vi "labview.vi"() -> ()   [LabVIEW 2021]
uses:
  40da32ed-f428-4d30-ba7b-34cf0621b097.vi
  <vilib>/Utility/file.llb/Read Delimited Spreadsheet (string).vi
  <vilib>/Comparison/Less/Less Functor/Less Functor.lvclass
panel:
  out "Buys Cumputer":string
  out "output cluster":T1
  in  "file path (dialog if empty)":path
  in  "K Value":dbl
  in  "Query Instance":T2
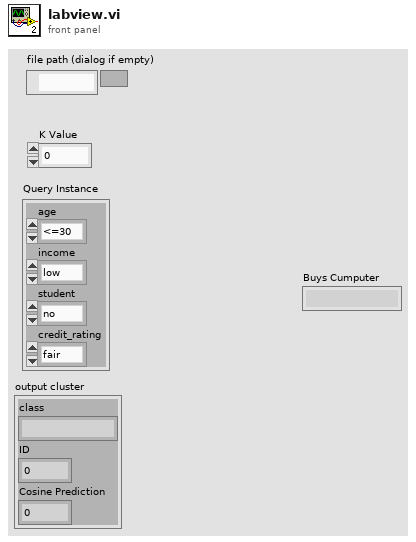
[diagram p1: front panel]
types:
  T1 = cluster{"class":string, "ID":dbl, "Cosine Prediction":dbl}
  T2 = cluster{"age":enum32{"<=30", "31...40", ">40"}, "income":enum32{"low", "medium", "high"}, "student":enum32{"no", "yes"}, "credit_rating":enum32{"fair", "excellent"}}
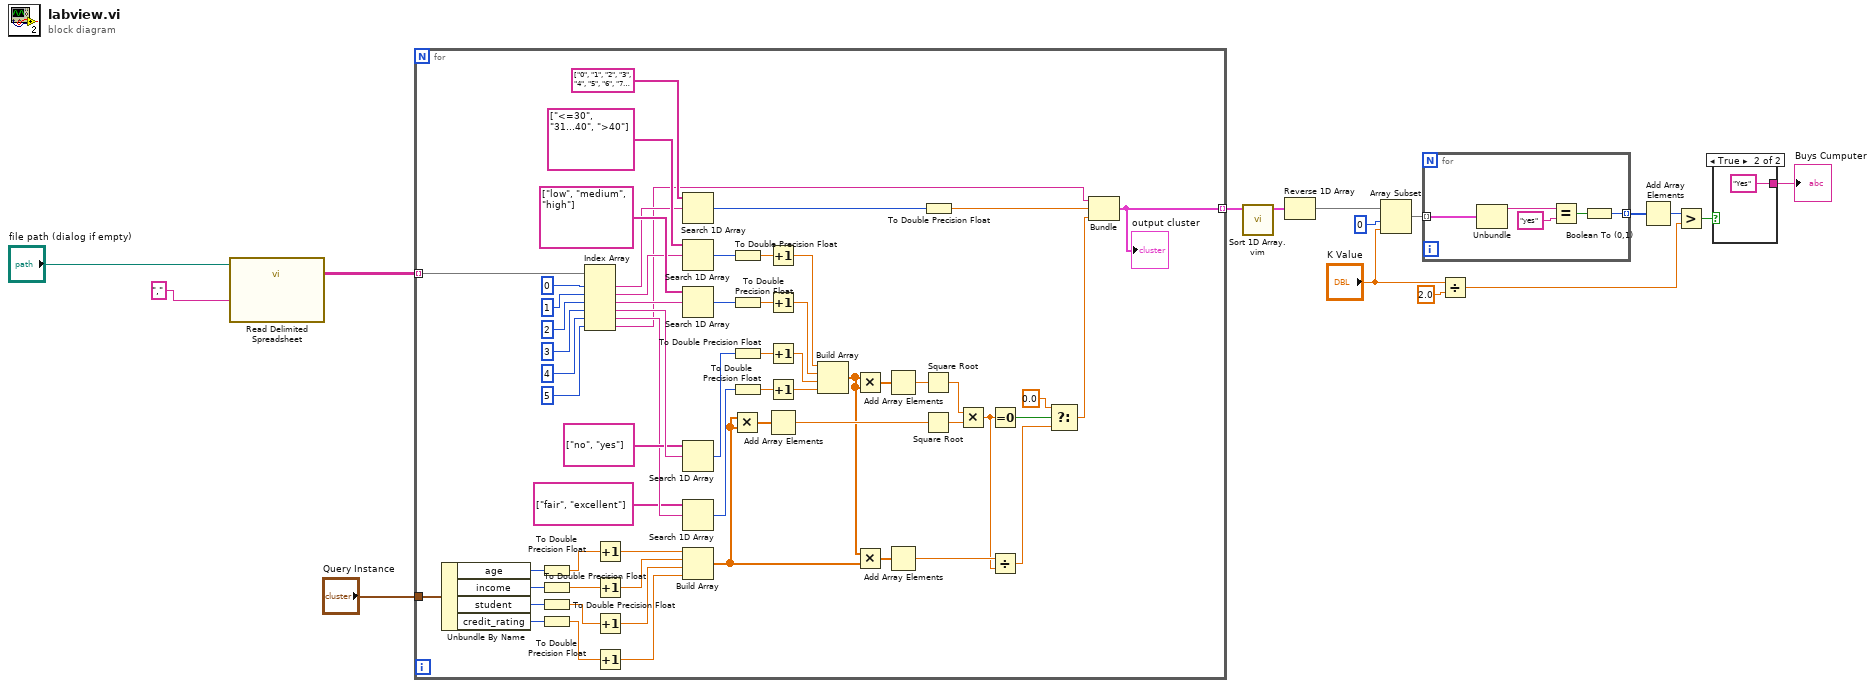
[diagram p0: block diagram]
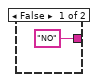
[diagram p2: hidden frame]
diagram:
  n1 = call-poly <vilib>:"Read Delimited Spreadsheet.vi"("file path (dialog if empty)"="file path (dialog if empty)", "delimiter (\\t)"="," ("delimiter (\\t)")) -> ("all rows"=w14:string[][])  [unwired: 8 in, 5 out]
  n2 = for {
    tunnel: w14 -> [w64] mode=indexing
    tunnel: "Query Instance" -> [w50]
    tunnel: [w24] -> w12 mode=indexing
    n3 = Unbundle By Name(w50) -> ("age"=w45:enum32{"<=30", "31...40", ">40"}, "income"=w44:enum32{"low", "medium", "high"}, "student"=w43:enum32{"no", "yes"}, "credit_rating"=w42:enum32{"fair", "excellent"})
    n4 = To Double Precision Float(number=w45) -> (double precision float=w49:dbl)
    n5 = To Double Precision Float(number=w44) -> (double precision float=w48:dbl)
    n6 = To Double Precision Float(number=w43) -> (double precision float=w47:dbl)
    n7 = To Double Precision Float(number=w42) -> (double precision float=w46:dbl)
    n8 = Index Array(array=w64, index #1=0 ("index"), index #2=1 ("index"), index #3=2 ("index"), index #4=3 ("index"), index #5=4 ("index"), index #6=5 ("index")) -> (element #1=w27:string, element #2=w70:string, element #3=w71:string, element #4=w68:string, element #5=w66:string, element #6=w18:string)
    n9 = Increment(x=w49) -> (x+1=w41:dbl)
    n10 = Increment(x=w48) -> (x+1=w40:dbl)
    n11 = Increment(x=w47) -> (x+1=w39:dbl)
    n12 = Increment(x=w46) -> (x+1=w38:dbl)
    n13 = Search 1D Array(1D array=string[] ["0", "1", "2", "3", "4", "5", "6", "7", "8", "9", "10", "11", "12", "13"], element=w27) -> (index of element=w26:i32)  [unwired: 1 in]
    n14 = Search 1D Array(1D array=string[] ["<=30", "31...40", ">40"], element=w70) -> (index of element=w62:i32)  [unwired: 1 in]
    n15 = Search 1D Array(1D array=string[] ["low", "medium", "high"], element=w71) -> (index of element=w59:i32)  [unwired: 1 in]
    n16 = Search 1D Array(1D array=string[] ["no", "yes"], element=w68) -> (index of element=w57:i32)  [unwired: 1 in]
    n17 = Search 1D Array(1D array=string[] ["fair", "excellent"], element=w66) -> (index of element=w55:i32)  [unwired: 1 in]
    n18 = Build Array(w41, w40, w39, w38) -> (w35:dbl[])
    n19 = Multiply(x=w35, y=w35) -> (x*y=w34:dbl[])
    n20 = To Double Precision Float(number=w62) -> (double precision float=w61:dbl)
    n21 = To Double Precision Float(number=w59) -> (double precision float=w60:dbl)
    n22 = To Double Precision Float(number=w57) -> (double precision float=w58:dbl)
    n23 = To Double Precision Float(number=w55) -> (double precision float=w56:dbl)
    n24 = Increment(x=w61) -> (x+1=w54:dbl)
    n25 = Increment(x=w60) -> (x+1=w53:dbl)
    n26 = Increment(x=w58) -> (x+1=w52:dbl)
    n27 = Increment(x=w56) -> (x+1=w51:dbl)
    n28 = Add Array Elements(numeric array=w34) -> (sum=w33:dbl)
    n29 = Build Array(w54, w53, w52, w51) -> (w29:dbl[])
    n30 = Multiply(x=w29, y=w29) -> (x*y=w32:dbl[])
    n31 = Multiply(x=w29, y=w35) -> (x*y=w37:dbl[])
    n32 = Add Array Elements(numeric array=w32) -> (sum=w31:dbl)
    n33 = Add Array Elements(numeric array=w37) -> (sum=w36:dbl)
    n34 = Square Root(x=w31) -> (sqrt(x)=w28:dbl)
    n35 = Square Root(x=w33) -> (sqrt(x)=w30:dbl)
    n36 = To Double Precision Float(number=w26) -> (double precision float=w17:dbl)
    n37 = Multiply(x=w28, y=w30) -> (x*y=w23:dbl)
    n38 = Equal To 0?(x=w23) -> (x = 0?=w22:bool)
    n39 = Divide(x=w36, y=w23) -> (x/y=w20:dbl)
    n40 = Select(t=0.0, s=w22, f=w20) -> (s? t:f=w19:dbl)
    n41 = Bundle("String"=w18, w17, "t"=w19) -> (w24:cluster{"String":string, dbl, "t":dbl})  [unwired: 1 in]
    "output cluster" <- w24
  }
  n42 = call "Sort 1D Array.vim"("unsorted array"=w12) -> ("sorted array"=w11:cluster{"String":string, dbl, "t":dbl}[])  [unwired: 10 in]
  n43 = Reverse 1D Array(array=w11) -> (reversed array=w10:cluster{"String":string, dbl, "t":dbl}[])
  n44 = Array Subset(array=w10, index=0, length="K Value") -> (w8:cluster{"String":string, dbl, "t":dbl}[])
  n45 = for {
    tunnel: w8 -> [w82] mode=indexing
    tunnel: [w78] -> w7 mode=indexing
    n46 = Unbundle(w82) -> ("String"=w80:string)  [unwired: 2 out]
    n47 = Equal?(x=w80, y="yes") -> (x = y?=w79:bool)
    n48 = Boolean To (0,1)(Boolean=w79) -> (0, 1=w78:i16)
  }
  n49 = Divide(x="K Value", y=2.0) -> (x/y=w3:dbl)
  n50 = Add Array Elements(numeric array=w7) -> (sum=w6:i16)
  n51 = Greater?(x=w6, y=w3) -> (0:w2:bool)
  n52 = case shown="True" w2 {
    tunnel: ["NO" "Yes"] -> w1
    frame False {
    }
    frame True {
    }
  }
  "Buys Cumputer" <- w1
